vi "Write Statistcs.vi"(8 "error in (no error)":errorcluster, 10 "Statistcs":T1, 11 "CAN_RW_CORE in":refnum<class "L2ENET_RW_CORE.lvclass">) -> (0 "error out":errorcluster, 3 "CAN_RW_CORE out":refnum<class "L2ENET_RW_CORE.lvclass">)   [LabVIEW 2021, in "L2ENET_RW_CORE.lvclass"]
uses:
  L2ENET_RW_CORE.lvclass
  L2ENET_RW_CORE.lvclass/L2ENET_RW_CORE.ctl
  typedef/Statistics.ctl
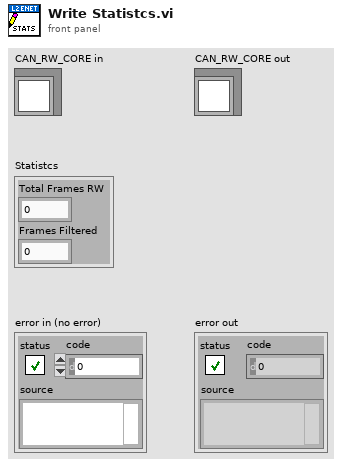
[diagram p1: front panel]
types:
  T1 = typedef "L2ENET_RW_CORE.lvclass/Statistics.ctl" = cluster{"Total Frames RW":u32, "Frames Filtered ":u32}
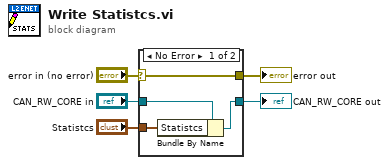
[diagram p0: block diagram]
diagram:
  n1 = case shown="No Error" "error in (no error)" {
    selector: "error in (no error)" -> [w9 w10]
    tunnel: [w9 w10] -> w4
    tunnel: [w7 w11] -> w2
    tunnel: "CAN_RW_CORE in" -> [w8 w11]
    tunnel: "Statistcs" -> [w6 _]
    frame No Error {
      n2 = Bundle By Name(cluster=w8, "Statistcs"=w6) -> (w7:refnum<class "L2ENET_RW_CORE.lvclass">)
    }
    frame Error {
    }
  }
  "error out" <- w4
  "CAN_RW_CORE out" <- w2
